vi "CameraStartAcquire.vi"(8 "error in (no error)":errorcluster, 11 "AndorSDK3 in":refnum<class "Andor3.lvclass">) -> (0 "error out":errorcluster, 3 "AndorSDK3 out":refnum<class "Andor3.lvclass">)   [LabVIEW 2010, in "Andor3.lvclass"]
uses:
  Andor3.lvclass
  Andor3.lvclass/Andor3.ctl
  <userlib>/atcoreA/atcoreA.lvlib
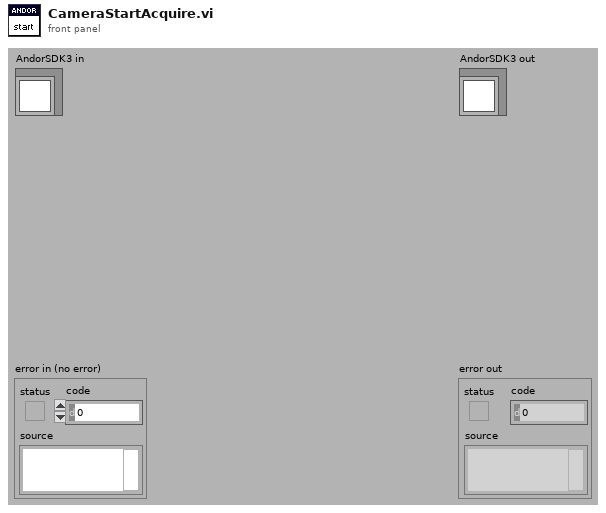
[diagram p1: front panel]
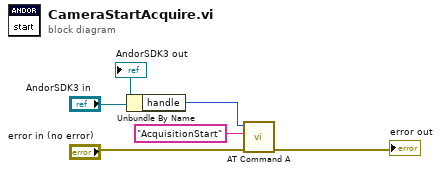
[diagram p0: block diagram]
diagram:
  n1 = Unbundle By Name("AndorSDK3 in") -> ("handle"=w2:i32)
  n2 = call <userlib>:"AT Command A.vi"("error in (no error)"="error in (no error)", "Feature"="AcquisitionStart", "Hndl"=w2) -> ("error out"=→"error out":errorcluster)  [unwired: 8 in]
  "AndorSDK3 out" <- "AndorSDK3 in"
